vi "UseClass - Reentrant.vi"() -> (3 "myClass.lvclass":refnum<class "MyClass - Reentrant.lvclass">)   [LabVIEW 2010]
uses:
  MyClass - Reentrant.lvclass
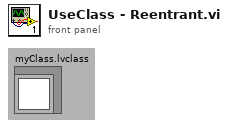
[diagram p1: front panel]
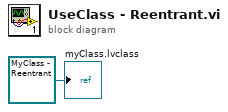
[diagram p0: block diagram]
diagram:
  "myClass.lvclass" <- refnum<class "MyClass - Reentrant.lvclass"> refnum ("myClass.lvclass")
